vi "2-1.vi"(1 "B":dbl, 2 "X":dbl, 3 "K":dbl) -> (0 "Y":dbl)   [LabVIEW 2017]
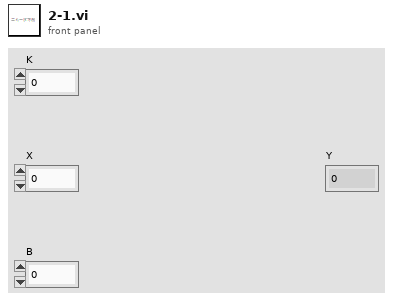
[diagram p1: front panel]
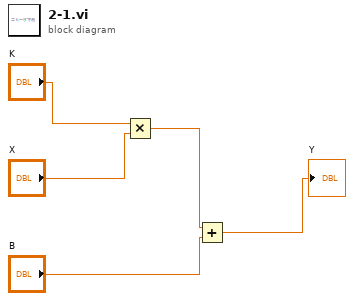
[diagram p0: block diagram]
diagram:
  n1 = Multiply(x="K", y="X") -> (x*y=w3:dbl)
  n2 = Add(x=w3, y="B") -> (x+y=→"Y":dbl)
